vi "PfeifferMVP15.vi"(6 "On?":bool, 7 "Write?":bool, 8 "error in":errorcluster, 9 "Cmd":T1, 10 "Adress":u16=1 max=999 step=1, 11 "VISA session":refnum<visa-resource-name>) -> (0 "error out":errorcluster, 2 "Result":variant, 3 "VISA session Out":refnum<visa-resource-name>)   [LabVIEW 2019]
uses:
  PfeifferMVP15Cmds.ctl
  <instrlib>/Pfeiffer Vacuum/Pfeiffer Vacuum.lvlib
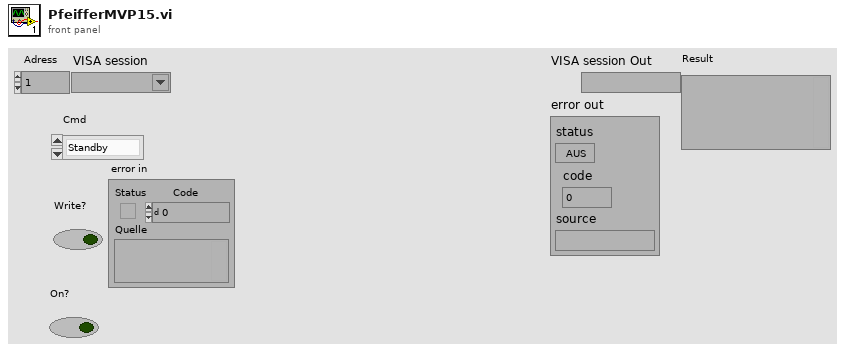
[diagram p1: front panel]
types:
  T1 = typedef "PfeifferMVP15Cmds.ctl" = enum16{"Standby", "Run", "AckError", "ErrorCode", "ActualSpdHz", "DrvCurrent", "OpHrsPump", "FwVersion", "DrvVoltage", "NominalSpdHz", "DrvPower", "ElecName", "HWVersion", "ActualSpdRPM", "NominalSpdRPM", "TempPump"}
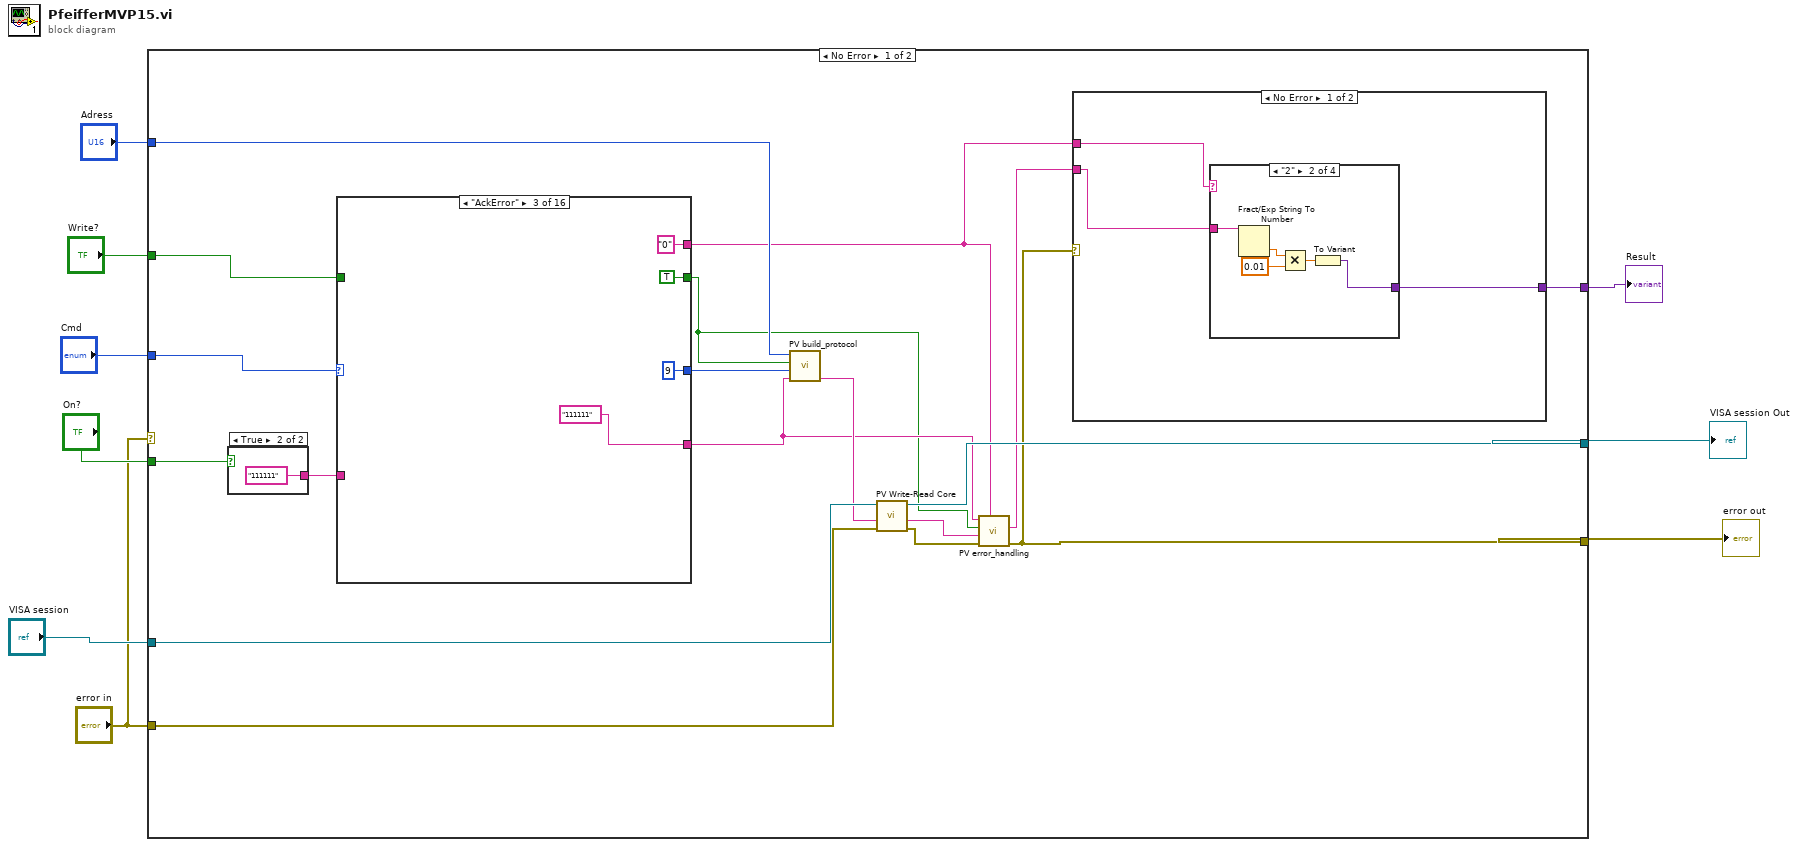
[diagram p0: block diagram]
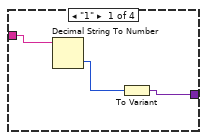
[diagram p2: hidden frame]
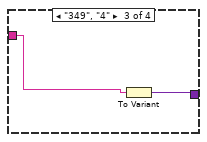
[diagram p3: hidden frame]
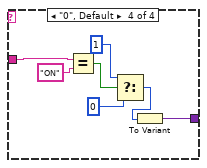
[diagram p4: hidden frame]
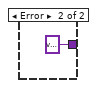
[diagram p5: hidden frame]
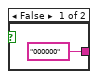
[diagram p6: hidden frame]
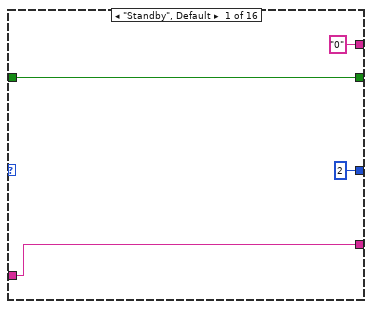
[diagram p7: hidden frame]
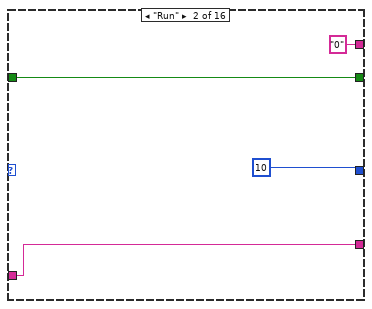
[diagram p8: hidden frame]
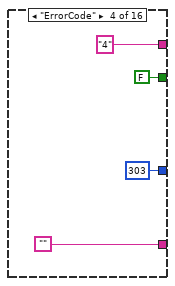
[diagram p9: hidden frame]
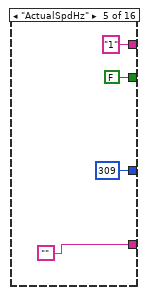
[diagram p10: hidden frame]
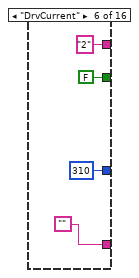
[diagram p11: hidden frame]
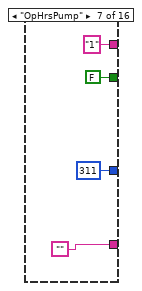
[diagram p12: hidden frame]
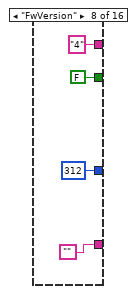
[diagram p13: hidden frame]
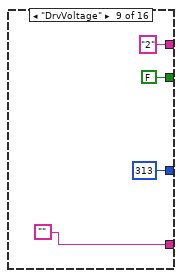
[diagram p14: hidden frame]
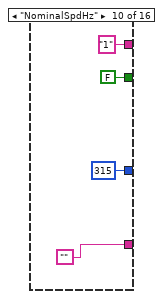
[diagram p15: hidden frame]
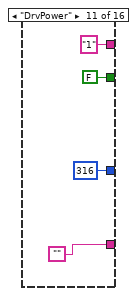
[diagram p16: hidden frame]
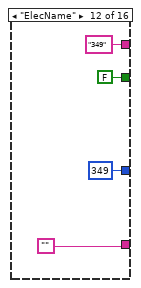
[diagram p17: hidden frame]
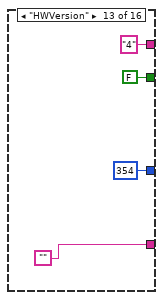
[diagram p18: hidden frame]
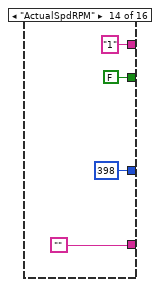
[diagram p19: hidden frame]
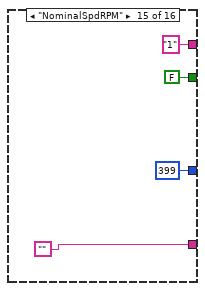
[diagram p20: hidden frame]
diagram:
  n1 = case shown="No Error" "error in" {
    tunnel: "Cmd" -> [w27 _]
    tunnel: "Adress" -> [w25 _]
    tunnel: "VISA session" -> [w24 w117]
    tunnel: [w23 w117] -> w6
    tunnel: "error in" -> [w21 w116]
    tunnel: "Write?" -> [w20 _]
    tunnel: [w13 w116] -> w4
    tunnel: "On?" -> [w15 _]
    tunnel: [w10 variant ("Variant")] -> w1
    frame No Error {
      n2 = case shown="True" w15 {
        tunnel: ["000000" ("Data") "111111" ("Data")] -> w14
        frame False {
        }
        frame True {
        }
      }
      n3 = case shown="\"AckError\"" w27 {
        tunnel: [u16 2 u16 10 u16 9 u16 303 u16 309 u16 310 u16 311 u16 312 u16 313 u16 315 u16 316 u16 349 u16 354 u16 398 u16 399 u16 330] -> w26
        tunnel: w20 -> [w54 w57 _ _ _ _ _ _ _ _ _ _ _ _ _ _]
        tunnel: [w54 w57 TRUE ("Write?") FALSE ("Write?") FALSE ("Write?") FALSE ("Write?") FALSE ("Write?") FALSE ("Write?") FALSE ("Write?") FALSE ("Write?") FALSE ("Write?") FALSE ("Write?") FALSE ("Write?") FALSE ("Write?") FALSE ("Write?") FALSE ("Write?")] -> w16
        tunnel: [w51 w55 "111111" ("Data") "" "" "" "" "" "" "" "" "" "" "" "" ""] -> w17
        tunnel: ["0" "0" "0" "4" "1" "2" "1" "4" "2" "1" "1" "349" "4" "1" "1" "1"] -> w11
        tunnel: w14 -> [w51 w55 _ _ _ _ _ _ _ _ _ _ _ _ _ _]
        frame "Standby", Default {
        }
        frame "Run" {
        }
        frame "AckError" {
        }
        frame "ErrorCode" {
        }
        frame "ActualSpdHz" {
        }
        frame "DrvCurrent" {
        }
        frame "OpHrsPump" {
        }
        frame "FwVersion" {
        }
        frame "DrvVoltage" {
        }
        frame "NominalSpdHz" {
        }
        frame "DrvPower" {
        }
        frame "ElecName" {
        }
        frame "HWVersion" {
        }
        frame "ActualSpdRPM" {
        }
        frame "NominalSpdRPM" {
        }
        frame "TempPump" {
        }
      }
      n4 = call <instrlib>:"PV build_protocol.vi"("Data"=w17, "Parameter-number"=w26, "parameter\nread<->describe"=w16, "Adress"=w25) -> ("output"=w22:string)  [unwired: 3 in]
      n5 = call <instrlib>:"PV Write-Read Core.vi"("error in"=w21, "Write data in"=w22, "VISA session"=w24) -> ("error out"=w19:errorcluster, "response (data) out"=w18:string, "dup VISA session"=w23:refnum<visa-resource-name>)  [unwired: 2 in]
      n6 = call <instrlib>:"PV error_handling.vi"("Data Typ in"=w11, "error in"=w19, "response (data) in"=w18, "Parameter\nread only<->describe"=w16, "data in"=w17) -> ("error out"=w13:errorcluster, "Data out"=w12:string)  [unwired: 4 in, 1 out]
      n7 = case shown="No Error" w13 {
        tunnel: w12 -> [w30 _]
        tunnel: w11 -> [w29 _]
        tunnel: [w28 variant ("Variant")] -> w10
        frame No Error {
          n8 = case shown="\"2\"" w29 {
            tunnel: w30 -> [w33 w38 w40 w42]
            tunnel: [w31 w34 w39 w45] -> w28
            frame "1" {
              n9 = Decimal String To Number(string=w33) -> (number=w32:i32)  [unwired: 2 in, 1 out]
              n10 = To Variant(anything=w32) -> (Variant=w31:variant)
            }
            frame "2" {
              n11 = Fract/Exp String To Number(string=w38) -> (number=w37:dbl)  [unwired: 3 in, 1 out]
              n12 = Multiply(x=w37, y=0.01) -> (x*y=w35:dbl)
              n13 = To Variant(anything=w35) -> (Variant=w34:variant)
            }
            frame "349", "4" {
              n14 = To Variant(anything=w40) -> (Variant=w39:variant)
            }
            frame "0", Default {
              n15 = Equal?(x=w42, y="ON") -> (x = y?=w41:bool)
              n16 = Select(t=1, s=w41, f=0) -> (s? t:f=w46:i32)
              n17 = To Variant(anything=w46) -> (Variant=w45:variant)
            }
          }
        }
        frame Error {
        }
      }
    }
    frame Error {
    }
  }
  "VISA session Out" <- w6
  "error out" <- w4
  "Result" <- w1
